vi "ReadCapacity.vi"(11 "POTTypedCircularBuffer in":refnum<class "ErrorLogBuffer.lvclass">) -> (2 "capacity":i32, 3 "POTTypedCircularBuffer out":refnum<class "ErrorLogBuffer.lvclass">)   [LabVIEW 2024, in "ErrorLogBuffer.lvclass"]
uses:
  ErrorLogBuffer.lvclass
  ErrorLogBuffer.lvclass/ErrorLogBuffer.ctl
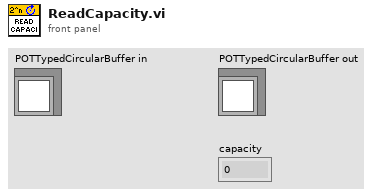
[diagram p1: front panel]
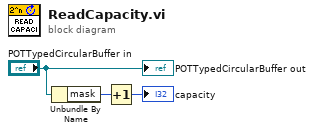
[diagram p0: block diagram]
diagram:
  n1 = Unbundle By Name("POTTypedCircularBuffer in") -> ("mask"=w2:i32)
  n2 = Increment(x=w2) -> (x+1=→"capacity":i32)
  "POTTypedCircularBuffer out" <- "POTTypedCircularBuffer in"
